vi "killtask-exe.vi"(8 "error in (no error)":errorcluster caption="错误输入（无错误）") -> (0 "error out":errorcluster caption="错误输出")   [LabVIEW 2013]
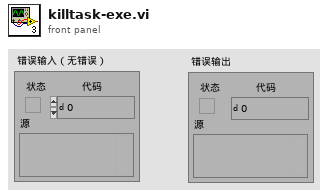
[diagram p1: front panel]
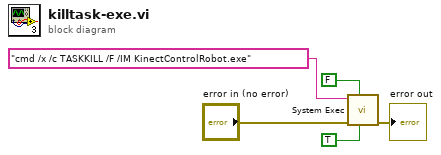
[diagram p0: block diagram]
diagram:
  n1 = call <vilib>:"System Exec.vi"("run minimized? (F)"=TRUE, "wait until completion? (T)"=FALSE ("Wait until done"), "error in (no error)"="error in (no error)", "command line"="cmd /x /c TASKKILL /F /IM KinectControlRobot.exe") -> ("error out"=→"error out":errorcluster)  [unwired: 2 in, 5 out]
